vi "Requests.vi"(8 "error in (no error)":errorcluster, 9 "write enable":bool=TRUE, 11 "ICPCON M-7024 in":refnum<class "ICPCON M-7024.lvclass">) -> (0 "error out":errorcluster, 3 "ICPCON M-7024 out":refnum<class "ICPCON M-7024.lvclass">)   [LabVIEW 2021, in "ICPCON M-7024.lvclass"]
uses:
  ICPCON M-7024.lvclass
  D:/my_projects/projects/Algorithms/Labview/21/Master CR/Master CR.lvclass
  D:/my_projects/projects/Algorithms/Labview/21/Master CR/Devices/Serial/Serial.lvclass
  Master CR.lvclass/Master CR.ctl
  Modbus_v121c/Modbus Data Unit/Modbus Data Unit.lvclass/Modbus Data Unit.ctl
  Modbus_v121c/Network Protocol/Network Master/Network Master.lvclass/Network Master.ctl
  Network Protocol/Read Network Protocol.vi
  Modbus_v121c/Master Function Definition/Read Holding Registers Request.vi
  Modbus_v121c/Master Function Definition/Read Holding Registers Response.vi
  Modbus_v121c/Network Protocol/Network Master/Read write Master.vi
  Modbus_v121c/Master Function Definition/Write Multiple Registers Request.vi
  Modbus_v121c/Master Function Definition/Function data mismatch error.vi
  Modbus_v121c/Master Function Definition/Write Multiple Registers Response.vi
  Modbus_v121c/Modbus Data Unit/Construct PDU.vi
  Modbus_v121c/Utility/Bytes to U16s.vi
  Modbus_v121c/Master Function Definition/Function code mismatch error.vi
  Modbus_v121c/Data Model/Error Generator.vi
  Modbus_v121c/Modbus Data Unit/Deconstruct PDU.vi
  Modbus_v121c/Utility/U16s to Bytes.vi
  Serial/Serial.lvclass
  Modbus_v121c/Network Protocol/Network Master/Network Master.lvclass
  Modbus_v121c/Modbus Data Unit/Modbus Data Unit.lvclass
  Modbus_v121c/Data Model/Device Data Model.lvclass
  Modbus_v121c/Transmission Data Unit/Transmission Data Unit.lvclass
  Master CR.lvclass
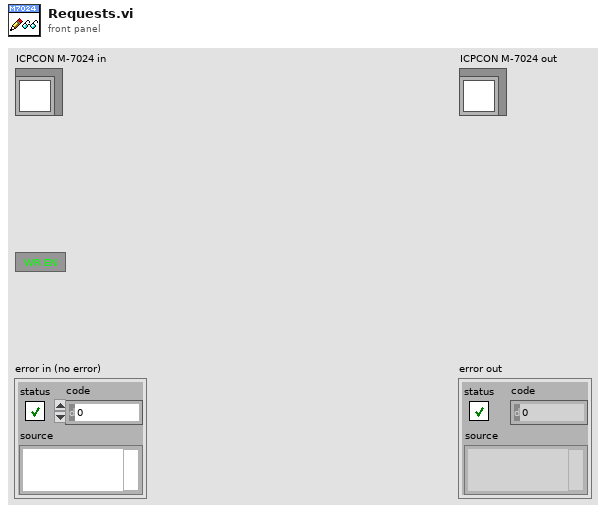
[diagram p1: front panel]
types:
  T1 = typedef "Device Data Model.lvclass/N channel.ctl" = cluster{"N DI channel":i32, "N DO channel":i32, "N AI channel":i32, "N AO channel":i32}
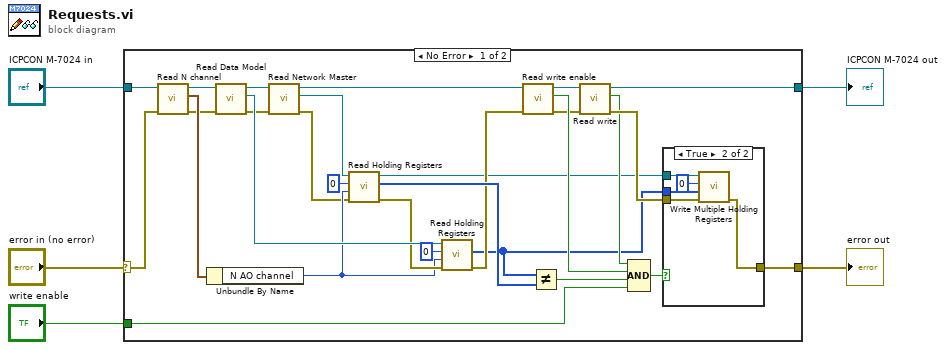
[diagram p0: block diagram]
diagram:
  n1 = case shown="No Error" "error in (no error)" {
    selector: "error in (no error)" -> [w29 w42]
    tunnel: [w33 w42] -> w3
    tunnel: [w12 w41] -> w4
    tunnel: "ICPCON M-7024 in" -> [w31 w41]
    tunnel: "write enable" -> [w25 _]
    frame No Error {
      n2 = call "Read N channel.vi"("error in (no error)"=w29, "Master CR in"=w31) -> ("error out"=w28:errorcluster, "N channel"=w32:T1, "Master CR out"=w30:refnum<class "ICPCON M-7024.lvclass">)  [unwired: 7 in]
      n3 = Unbundle By Name(w32) -> ("N AO channel"=w15:i32)
      n4 = call "Read Data Model.vi"("error in (no error)"=w28, "Master CR in"=w30) -> ("error out"=w9:errorcluster, "Data Model"=w20:refnum<class "Device Data Model.lvclass">, "Master CR out"=w10:refnum<class "ICPCON M-7024.lvclass">)  [unwired: 7 in]
      n5 = call "Read Network Master.vi"("error in (no error)"=w9, "Serial in"=w10) -> ("error out"=w7:errorcluster, "Network Master"=w6:refnum<class "Network Master.lvclass">, "Serial out"=w8:refnum<class "ICPCON M-7024.lvclass">)  [unwired: 7 in]
      n6 = call "Read Holding Registers.vi"("error in (no error)"=w7, "number of holding registers"=w15, "starting address"=u16 0, "Modbus master in"=w6) -> ("error out"=w16:errorcluster, "register values"=w18:u16[], "Modbus master out"=w11:refnum<class "Network Master.lvclass">)  [unwired: 5 in]
      n7 = call-dynamic "Read Holding Registers.vi"("error in"=w16, "number of registers"=w15, "starting address"=u16 0, "device data model in"=w20) -> ("error out"=w17:errorcluster, "data"=w14:u16[])  [unwired: 5 in, 1 out]
      n8 = call "Read write enable.vi"("error in (no error)"=w17, "Master CR in"=w8) -> ("error out"=w24:errorcluster, "write enable"=w26:bool, "Master CR out"=w13:refnum<class "ICPCON M-7024.lvclass">)  [unwired: 7 in]
      n9 = Not Equal?(x=w14, y=w18) -> (x != y?=w27:bool)
      n10 = call "Read write.vi"("error in (no error)"=w24, "Master CR in"=w13) -> ("error out"=w23:errorcluster, "Write"=w22:bool, "Master CR out"=w12:refnum<class "ICPCON M-7024.lvclass">)  [unwired: 7 in]
      n11 = Compound Arithmetic op=AND(w22, w26, w27, w25) -> (w34:bool)
      n12 = case shown="True" w34 {
        tunnel: w23 -> [w35 w39]
        tunnel: [w35 w37] -> w33
        tunnel: w14 -> [_ w38]
        tunnel: w11 -> [_ w36]
        frame False {
        }
        frame True {
          n13 = call "Write Multiple Holding Registers.vi"("error in (no error)"=w39, "holding register values"=w38, "starting address"=u16 0, "Modbus master in"=w36) -> ("error out"=w37:errorcluster)  [unwired: 6 in, 1 out]
        }
      }
    }
    frame Error {
    }
  }
  "error out" <- w3
  "ICPCON M-7024 out" <- w4
